vi "LanceurTempo&TrigSARAH.vi"(4 "entrée d'erreur (pas d'erreur)":errorcluster, 5 "Tempo Mes-Largage (ms)":i32=5000, 6 "Tempo Houle - Mes (ms)":i32=5000, 7 "task in":refnum<k21>) -> (0 "sortie d'erreur":errorcluster)   [LabVIEW 2017]
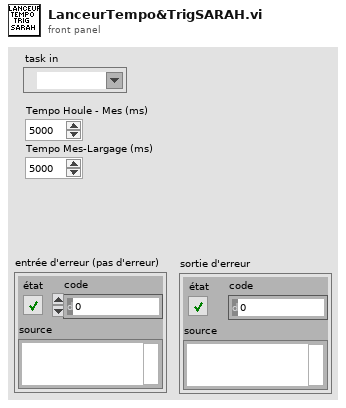
[diagram p1: front panel]
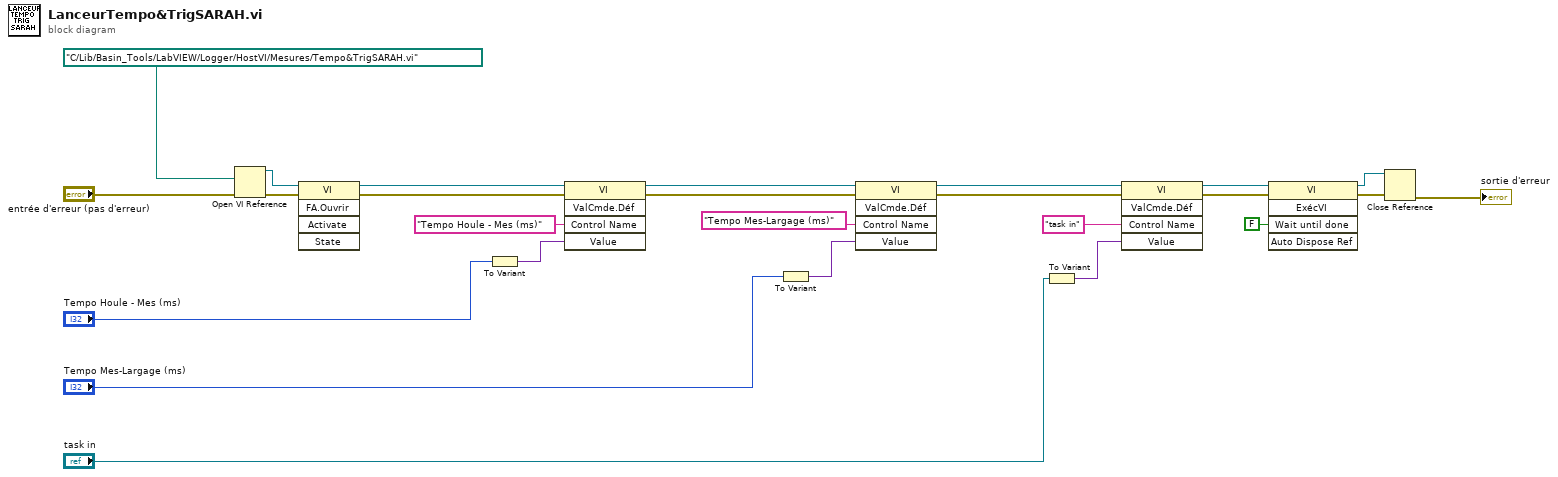
[diagram p0: block diagram]
diagram:
  n1 = Open VI Reference(vi path=path "C:/Lib/Basin_Tools/LabVIEW/Logger/HostVI/Mesures/Tempo&TrigSARAH.vi" ("chemin du VI"), error in (no error)="entrée d'erreur (pas d'erreur)") -> (vi reference=w22:refnum<vi>, error out=w21:errorcluster)  [unwired: 4 in]
  n2 = invoke class="VI" method="FA.Ouvrir"(reference=w22, error in=w21) -> (reference out=w19:refnum<vi>, error out=w18:errorcluster)  [unwired: 3 in, 3 out]
  n3 = To Variant(anything="Tempo Houle - Mes (ms)") -> (Variant=w15:variant)
  n4 = invoke class="VI" method="ValCmde.Déf"(reference=w19, error in=w18, "Control Name"="Tempo Houle - Mes (ms)" ("Nom de la commande"), "Value"=w15) -> (reference out=w11:refnum<vi>, error out=w10:errorcluster)  [unwired: 1 in, 3 out]
  n5 = To Variant(anything="Tempo Mes-Largage (ms)") -> (Variant=w14:variant)
  n6 = invoke class="VI" method="ValCmde.Déf"(reference=w11, error in=w10, "Control Name"="Tempo Mes-Largage (ms)" ("Nom de la commande"), "Value"=w14) -> (reference out=w5:refnum<vi>, error out=w4:errorcluster)  [unwired: 1 in, 3 out]
  n7 = To Variant(anything="task in") -> (Variant=w6:variant)
  n8 = invoke class="VI" method="ValCmde.Déf"(reference=w5, error in=w4, "Control Name"="task in" ("Nom de la commande"), "Value"=w6) -> (reference out=w3:refnum<vi>, error out=w2:errorcluster)  [unwired: 1 in, 3 out]
  n9 = invoke class="VI" method="ExécVI"(reference=w3, error in=w2, "Wait until done"=FALSE ("Attendre la fin")) -> (reference out=w23:refnum<vi>, error out=w24:errorcluster)  [unwired: 2 in, 3 out]
  n10 = Close Reference(reference=w23, error in (no error)=w24) -> (error out=→"sortie d'erreur":errorcluster)
